vi "float_precision.vi"(0 "input":dbl=22.2826 format="%#.12f", 1 "precision":i32=3) -> (2 "string":string)   [LabVIEW 2019, in "Tools.lvlib"]
uses:
  Tools.lvlib
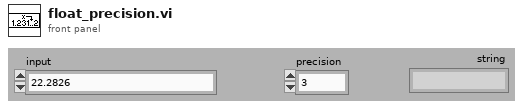
[diagram p1: front panel]
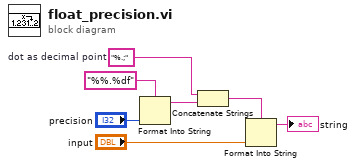
[diagram p0: block diagram]
diagram:
  w1 = "%.;"  # dot as decimal point
  n1 = Format Into String(format string="%%.%df", "precision") -> (resulting string=w6:string)  [unwired: 2 in, 1 out]
  n2 = Concatenate Strings(w1, w6) -> (w2:string)
  n3 = Format Into String(format string=w2, "input") -> (resulting string=→"string":string)  [unwired: 2 in, 1 out]
